vi "ErrorHandlerEventLoop.vi"(0 "object in":refnum<class "Application.lvclass">, 5 "error in (no error)":errorcluster) -> (14 "object out":refnum<class "Application.lvclass">, 19 "error out":errorcluster)   [LabVIEW 2021, in "Application.lvclass"]
uses:
  Application.lvclass
panel:
  in  "Ignore Errors (Runtime)":i32[](array[numeric])
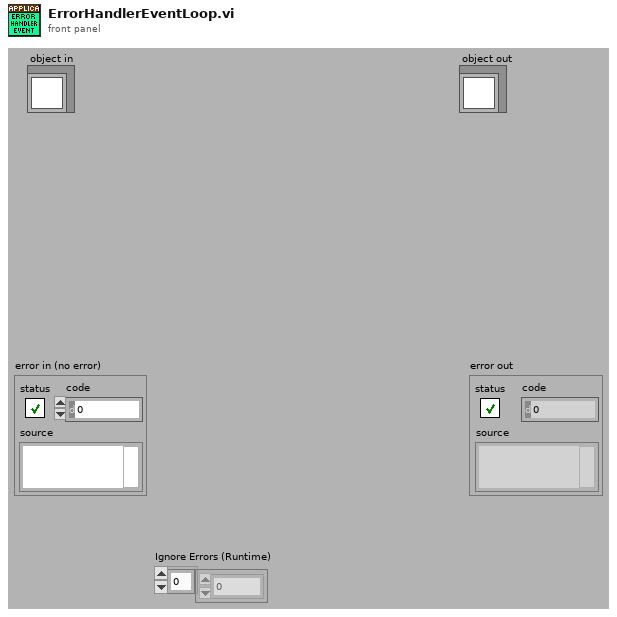
[diagram p1: front panel]
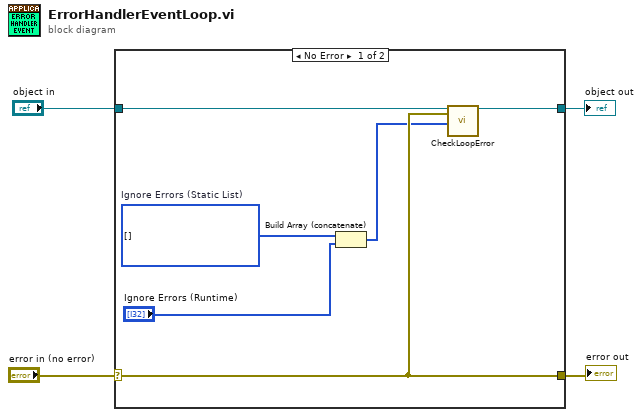
[diagram p0: block diagram]
diagram:
  n1 = case shown="No Error" "error in (no error)" {
    selector: "error in (no error)" -> [w6 w12]
    tunnel: [w6 w12] -> w3
    tunnel: [w8 w11] -> w1
    tunnel: "object in" -> [w7 w11]
    frame No Error {
      w10 = i32[] []  # Ignore Errors (Static List)
      n2 = Build Array (concatenate)(w10, "Ignore Errors (Runtime)") -> (w5:i32[])
      n3 = call-dynamic "CheckLoopError.vi"("object in"=w7, "error to process"=w6, "Ignore Errors"=w5) -> ("object out"=w8:refnum<class "Application.lvclass">)  [unwired: 15 in, 1 out]
    }
    frame Error {
    }
  }
  "error out" <- w3
  "object out" <- w1
